vi "Test.vi"(8 "error in (no error)":errorcluster, 11 "FTP in":refnum<class "FTP.lvclass">) -> (0 "error out":errorcluster)   [LabVIEW 2020, in "FTP.lvlib" / "FTP.lvclass"]
uses:
  FTP.lvclass
  controls/Dir-File Info.ctl
  controls/Dir-File Type.ctl
panel:
  out "Dir-File Info Array 2":T1[](array[typedef])
  out "Slide":u8(slide) scale=0.0..100.0
  out "Dir-File Info Array":T1[](array[typedef])
  out "time stamp":timestamp
  out "FileSize":i64
  out "cmdStrings":string
  in  "Local FilePath":path=path "C:/Users/jgoldberg.EVALUMATION/Desktop/adcConv.m"
  out "Current Directory":string
  in  "passWord":string
  in  "userName":string
  in  "address":string
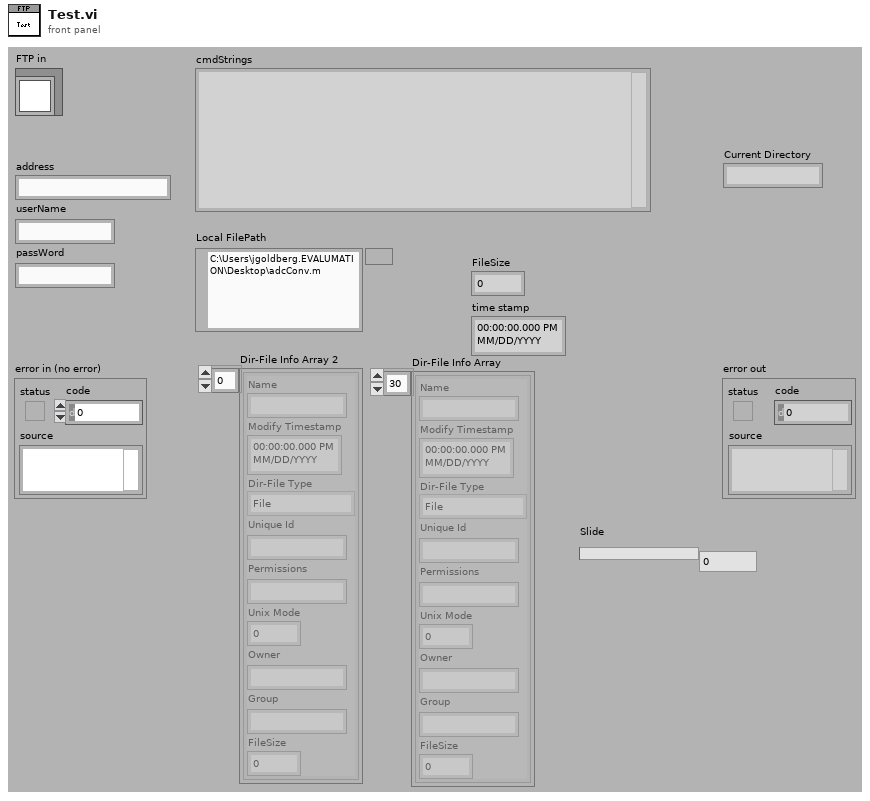
[diagram p1: front panel]
types:
  T1 = typedef "FTP.lvlib/FTP.lvclass/Dir-File Info.ctl" = cluster{"Name":string, "Modify Timestamp":timestamp, "Dir-File Type":T2, "Unique Id":string, "Permissions":string, "Unix Mode":u16, "Owner":string, "Group":string, "FileSize":i64}
  T2 = typedef "FTP.lvlib/FTP.lvclass/Dir-File Type.ctl" = enum16{"File", "Listed Directory", "Parent Directory", "Directory", "Unknown"}
  T3 = typedef "CmdCluster.ctl" = cluster{"CmdSting":string, "FromClient":bool}
  T4 = typedef "FTP.lvclass/File Transfer Status.ctl" = cluster{"File Name":string, "Percent Complete":u8, "File Size (in bytes)":i64, "Bytes Sent or Rcvd":i64}
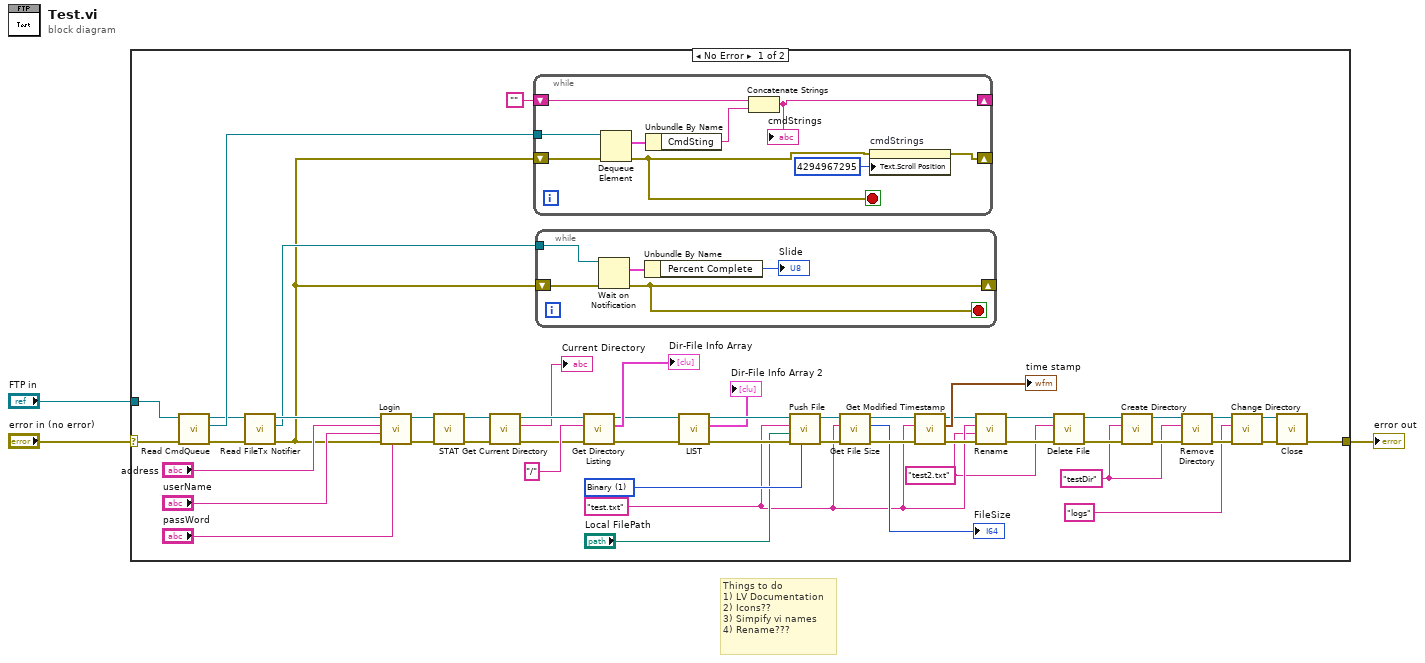
[diagram p0: block diagram]
diagram:
  # "Things to do\n1) LV Documentation\n2) Icons??\n3) Simpify vi names\n4) Rename???"
  n1 = case shown="No Error" "error in (no error)" {
    selector: "error in (no error)" -> [w24 w69]
    tunnel: [w54 w69] -> w2
    tunnel: "FTP in" -> [w23 _]
    frame No Error {
      w10 = "test2.txt" ("New FileName")
      w43 = "testDir" ("Remote Directory")
      w35 = u16 1 items=["ASCII", "Binary"] ("Type")
      w11 = "test.txt" ("FileName")
      n2 = call "Read CmdQueue.vi"("error in (no error)"=w24, "FTP in"=w23) -> ("error out"=w20:errorcluster, "CmdQueue"=w50:refnum<queue>, "FTP out"=w21:refnum<class "FTP.lvclass">)  [unwired: 7 in]
      n3 = call "Read FileTx Notifier.vi"("error in (no error)"=w20, "FTP in"=w21) -> ("error out"=w16:errorcluster, "FileTx Notifier"=w17:refnum<notifier>, "FTP out"=w19:refnum<class "FTP.lvclass">)  [unwired: 7 in]
      n4 = call "Login.vi"("passWord"="passWord", "error in (no error)"=w16, "userName"="userName", "address"="address", "FTP in"=w19) -> ("error out"=w18:errorcluster, "FTP out"=w22:refnum<class "FTP.lvclass">)  [unwired: 5 in]
      n5 = call "STAT.vi"("error in (no error)"=w18, "FTP in"=w22) -> ("error out"=w27:errorcluster, "FTP out"=w28:refnum<class "FTP.lvclass">)  [unwired: 7 in, 1 out]
      n6 = call "Get Current Directory.vi"("error in (no error)"=w27, "FTP in"=w28) -> ("error out"=w40:errorcluster, "Current Directory"=→"Current Directory":string, "FTP out"=w41:refnum<class "FTP.lvclass">)  [unwired: 7 in]
      n7 = while {
        tunnel: w50 -> [w68]
        shift-right: [w61] -> _
        shift-left: w16 -> [w67]
        shift-right: [w63] -> _
        shift-left: "" -> [w65]
        stop <- w60 stop-if-true
        n8 = Dequeue Element(queue=w68, error in (no error)=w67) -> (element=w66:T3, error out=w60:errorcluster)  [unwired: 1 in, 2 out]
        n9 = Unbundle By Name(w66) -> ("CmdSting"=w64:string)
        n10 = Concatenate Strings(w65, w64) -> (w63:string)
        "cmdStrings" <- w63
        n11 = property on="cmdStrings" class="Str"(error in=w60, "Text.Scroll Position"=u32 4294967295) -> (error out=w61:errorcluster)  [unwired: 1 in, 1 out]
      }
      n12 = while {
        tunnel: w17 -> [w58]
        shift-right: [w55] -> _
        shift-left: w16 -> [w59]
        stop <- w55 stop-if-true
        n13 = Wait on Notification(notifier=w58, error in (no error)=w59) -> (notification=w57:T4, error out=w55:errorcluster)  [unwired: 2 in, 2 out]
        n14 = Unbundle By Name(w57) -> ("Percent Complete"=→"Slide":u8)
      }
      n15 = call "Get Directory Listing.vi"("error in (no error)"=w40, "RemoteDirectory"="/", "FTP in"=w41) -> ("error out"=w25:errorcluster, "Dir-File Info Array"=→"Dir-File Info Array":T1[], "FTP out"=w26:refnum<class "FTP.lvclass">)  [unwired: 6 in]
      n16 = call "LIST.vi"("error in (no error)"=w25, "FTP in"=w26) -> ("error out"=w37:errorcluster, "Dir-File Info Array"=→"Dir-File Info Array 2":T1[], "FTP out"=w36:refnum<class "FTP.lvclass">)  [unwired: 7 in]
      n17 = call "Push File.vi"("Type (Binary)"=w35, "error in (no error)"=w37, "Local FilePath"="Local FilePath", "Remote FileName"=w11, "FTP in"=w36) -> ("error out"=w32:errorcluster, "FTP out"=w33:refnum<class "FTP.lvclass">)  [unwired: 5 in]
      n18 = call "Get File Size.vi"("error in (no error)"=w32, "Remote FileName"=w11, "FTP in"=w33) -> ("error out"=w30:errorcluster, "FileSize"=→"FileSize":i64, "FTP out"=w31:refnum<class "FTP.lvclass">)  [unwired: 6 in]
      n19 = call "Get Modified Timestamp.vi"("error in (no error)"=w30, "RemoteFileName"=w11, "FTP in"=w31) -> ("error out"=w15:errorcluster, "Modified Timestamp"=→"time stamp":timestamp, "FTP out"=w14:refnum<class "FTP.lvclass">)  [unwired: 6 in]
      n20 = call "Rename.vi"("error in (no error)"=w15, "New FileName"=w10, "File To Rename"=w11, "FTP in"=w14) -> ("error out"=w12:errorcluster, "FTP out"=w13:refnum<class "FTP.lvclass">)  [unwired: 6 in]
      n21 = call "Delete File.vi"("error in (no error)"=w12, "RemoteFileName"=w10, "FTP in"=w13) -> ("error out"=w47:errorcluster, "FTP out"=w46:refnum<class "FTP.lvclass">)  [unwired: 7 in]
      n22 = call "Create Directory.vi"("error in (no error)"=w47, "Remote Directory"=w43, "FTP in"=w46) -> ("error out"=w44:errorcluster, "FTP out"=w45:refnum<class "FTP.lvclass">)  [unwired: 7 in]
      n23 = call "Remove Directory.vi"("error in (no error)"=w44, "Remote Directory"=w43, "FTP in"=w45) -> ("error out"=w8:errorcluster, "FTP out"=w9:refnum<class "FTP.lvclass">)  [unwired: 7 in]
      n24 = call "Change Directory.vi"("error in (no error)"=w8, "RemoteDirectory"="logs" ("Remote Directory"), "FTP in"=w9) -> ("error out"=w6:errorcluster, "FTP out"=w7:refnum<class "FTP.lvclass">)  [unwired: 7 in]
      n25 = call "Close.vi"("error in (no error)"=w6, "FTP in"=w7) -> ("error out"=w54:errorcluster)  [unwired: 9 in]
    }
    frame Error {
    }
  }
  "error out" <- w2
